vi "Situation at Time t.vi"(6 "number of points":i32=64, 9 "flaws (circles)":cluster{"x0":dbl, "y0":dbl, "r":dbl}[](array[cluster]), 10 "y source":dbl, 11 "x source":dbl=1.0) -> (3 "tomography array":dbl[][](array[numeric]))   [LabVIEW 2023]
doc: "Calculate tomography array."
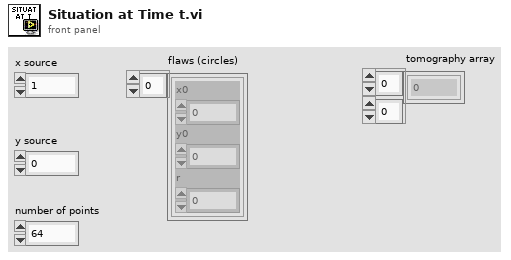
[diagram p1: front panel]
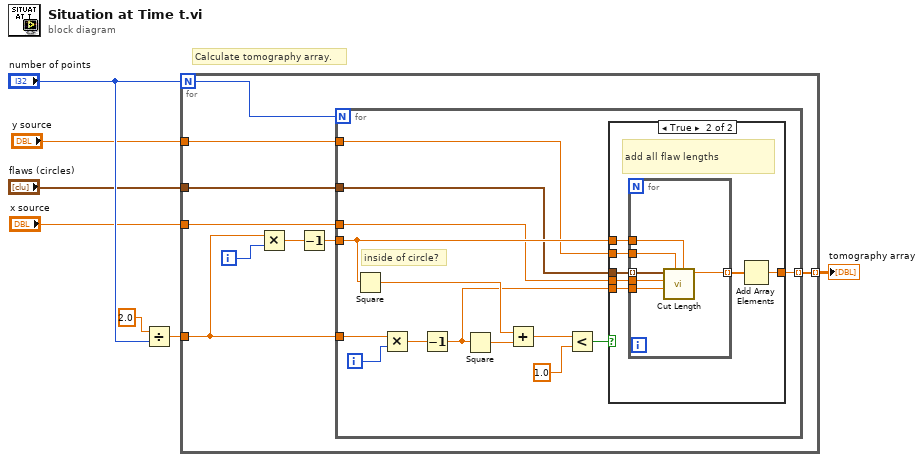
[diagram p0: block diagram]
diagram:
  # "Calculate tomography array."
  n1 = Divide(x=2.0, y="number of points") -> (x/y=w6:dbl)
  n2 = for {
    N: "number of points" -> [w11]
    tunnel: w6 -> [w15]
    tunnel: [w13] -> w5 mode=indexing
    tunnel: "flaws (circles)" -> [w12]
    tunnel: "y source" -> [w9]
    tunnel: "x source" -> [w8]
    i -> [w10]
    n3 = Multiply(x=w15, y=w10) -> (x*y=w16:dbl)
    n4 = Decrement(x=w16) -> (x-1=w14:dbl)
    n5 = for {
      N: w11 -> [_]
      tunnel: w15 -> [w30]
      tunnel: w14 -> [w23]
      tunnel: [w27] -> w13 mode=indexing
      tunnel: w12 -> [w20]
      tunnel: w9 -> [w18]
      tunnel: w8 -> [w17]
      i -> [w29]
      # "inside of circle?"
      n6 = Square(x=w23) -> (x^2=w26:dbl)
      n7 = Multiply(x=w30, y=w29) -> (x*y=w28:dbl)
      n8 = Decrement(x=w28) -> (x-1=w22:dbl)
      n9 = Square(x=w22) -> (x^2=w25:dbl)
      n10 = Add(x=w26, y=w25) -> (x+y=w24:dbl)
      n11 = Less?(x=w24, y=1.0) -> (x < y?=w21:bool)
      n12 = case shown="True" w21 {
        tunnel: w17 -> [_ w34]
        tunnel: w18 -> [_ w35]
        tunnel: w22 -> [_ w33]
        tunnel: w23 -> [_ w36]
        tunnel: [_ w31] -> w27
        tunnel: w20 -> [_ w37]
        frame False {
        }
        frame True {
          # "add all flaw lengths"
          n13 = for {
            tunnel: w37 -> [w43] mode=indexing
            tunnel: w36 -> [w42]
            tunnel: w35 -> [w41]
            tunnel: w34 -> [w39]
            tunnel: w33 -> [w38]
            tunnel: [w40] -> w32 mode=indexing
            n14 = call "Cut Length.vi"("y2"=w42, "y1"=w41, "x2"=w38, "x1"=w39, "circle"=w43) -> ("length"=w40:dbl)  [unwired: 6 in]
          }
          n15 = Add Array Elements(numeric array=w32) -> (sum=w31:dbl)
        }
      }
    }
  }
  "tomography array" <- w5
